vi "UI V7.1.3.vi"() -> ()   [LabVIEW 2017]
uses:
  <vilib>/Instr/_visa.llb/VISA Configure Serial Port (Instr).vi
  <vilib>/addons/Biomedical/Biosignal Measurements/Biosignal Preprocessing/Biosignal Rate Extractor (Waveform).vi
  <vilib>/addons/Biomedical/NI_BMTK_Measurements.lvlib
panel:
  out "CH2":u16(slide) scale=0.0..1000.0
  out "CH2 PM":dbl
  in  "Stop Button":bool
  out "led ch1 2":bool
  out "led ch1":bool
  out "CH1":u16(slide) scale=0.0..1000.0
  out "CH1 PM":dbl
  out "CH1":waveform(u16)(graph)
  out "CH2":waveform(u16)(graph)
  in  "?":refnum<visa-resource-name>
  # "HR and Respiration Counter V7.1.3"
  # "FEE BME | Menofia University"
  # "Made by \nNour Team"
  # "CH1"
  # "CH2"
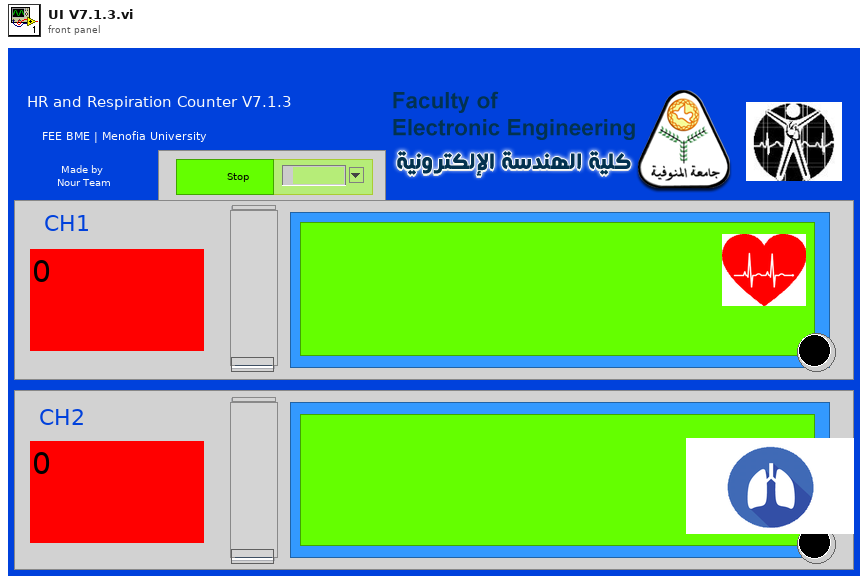
[diagram p1: front panel]
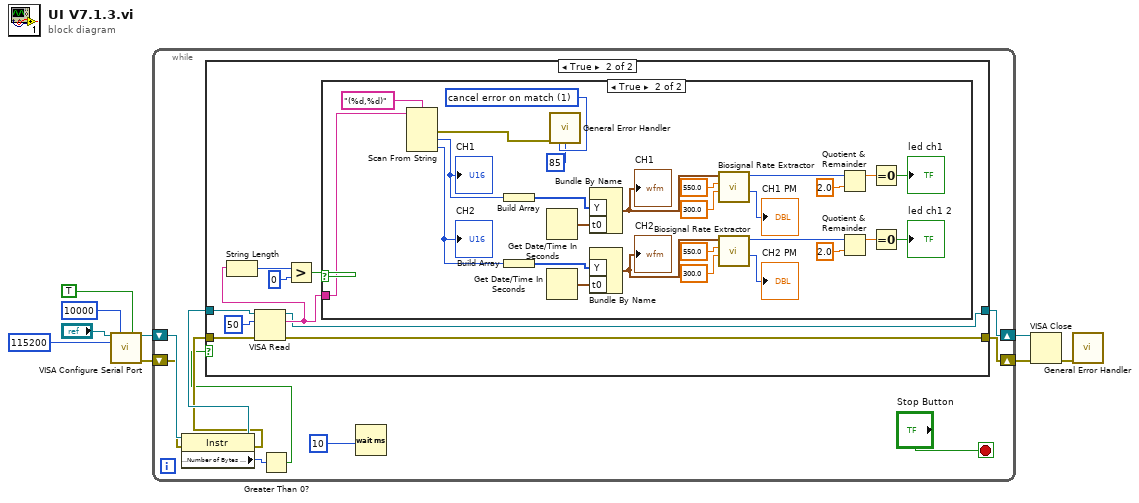
[diagram p0: block diagram]
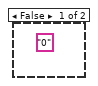
[diagram p3: hidden frame]
diagram:
  n1 = call-poly "VISA Configure Serial Port"("VISA resource name"="?", "timeout (10sec)"=u32 10000, "Enable Termination\nChar (T)"=TRUE ("Enable Termination\nChar (T)"), "baud rate (9600)"=u32 115200) -> ("VISA resource name out"=w2:refnum<visa-resource-name>, "error out"=w1:errorcluster)  [unwired: 10 in]
  n2 = while {
    shift-right: [w19] -> w7
    shift-left: w2 -> [w14]
    shift-right: [w12] -> w6
    shift-left: w1 -> [w13]
    stop <- "Stop Button" stop-if-true
    n3 = property class="Instr"(reference=w14, error in=w13) -> (reference out=w18:refnum<visa-resource-name>, error out=w17:errorcluster, "Serial Settings:Number of Bytes at Serial Port"=w16:u32)
    n4 = Greater Than 0?(x=w16) -> (x > 0?=w15:bool)
    n5 = case shown="True" w15 {
      tunnel: w18 -> [w21 w30]
      tunnel: w17 -> [w20 w29]
      tunnel: [w21 w24] -> w19
      tunnel: [w20 w23] -> w12
      frame False {
      }
      frame True {
        n6 = VISA Read(VISA resource name=w30, byte count=u32 50, error in (no error)=w29) -> (VISA resource name out=w24:refnum<visa-resource-name>, read buffer=w28:string, error out=w23:errorcluster)  [unwired: 1 out]
        n7 = String Length(string=w28) -> (length=w27:i32)
        n8 = Greater?(x=w27, y=0) -> (0:w25:bool)
        n9 = case shown="True" w25 {
          tunnel: w28 -> [_ w57]
          frame False {
            (unwired) "0"
          }
          frame True {
            w55 = 1 items=["no exception", "cancel error on match", "set error on match"] ("[exception action] (none:0)")
            n10 = Scan From String(format string="(%d,%d)", input string=w57) -> (error out=w54:errorcluster, output 1=w32:u16, output 2=w31:u16)  [unwired: 4 in, 2 out]
            "CH1" <- w32
            "CH2" <- w31
            n11 = Build Array(w32) -> (w33:u16[])
            n12 = Build Array(w31) -> (w44:u16[])
            n13 = Get Date/Time In Seconds() -> (seconds since 1Jan1904=w51:timestamp)
            n14 = Get Date/Time In Seconds() -> (seconds since 1Jan1904=w39:timestamp)
            n15 = call <vilib>:"General Error Handler.vi"("error in (no error)"=w54, "[exception action] (none:0)"=w55, "[exception code]"=85) -> ()  [unwired: 8 in, 5 out]
            n16 = Bundle By Name("Y"=w33, "t0"=w51) -> (w36:waveform(u16))  [unwired: 1 in]
            "CH1" <- w36
            n17 = Bundle By Name("Y"=w44, "t0"=w39) -> (w37:waveform(u16))  [unwired: 1 in]
            "CH2" <- w37
            n18 = call-poly <vilib>:"Biosignal Rate Extractor.vi"("low threshold"=300.0, "high threshold"=550.0, "biosignal"=w36) -> ("number of cycles per minuets"=→"CH1 PM":i32, "number of cycles"=w52:i32)  [unwired: 5 in, 2 out]
            n19 = call-poly <vilib>:"Biosignal Rate Extractor.vi"("low threshold"=300.0, "high threshold"=550.0, "biosignal"=w37) -> ("number of cycles per minuets"=→"CH2 PM":i32, "number of cycles"=w38:i32)  [unwired: 5 in, 2 out]
            n20 = Quotient & Remainder(x=w52, y=2.0) -> (x-y*floor(x/y)=w50:dbl)  [unwired: 1 out]
            n21 = Quotient & Remainder(x=w38, y=2.0) -> (x-y*floor(x/y)=w40:dbl)  [unwired: 1 out]
            n22 = Equal To 0?(x=w50) -> (x = 0?=→"led ch1":bool)
            n23 = Equal To 0?(x=w40) -> (x = 0?=→"led ch1 2":bool)
          }
        }
      }
    }
    n24 = Wait (ms)(milliseconds to wait=u32 10) -> ()  [unwired: 1 out]
  }
  n25 = VISA Close(VISA resource name=w7, error in (no error)=w6) -> (error out=w5:errorcluster)
  n26 = call <vilib>:"General Error Handler.vi"("error in (no error)"=w5) -> ()  [unwired: 10 in, 5 out]
